vi "initialize_oscilloscope_chan1.vi"(0 "Range (0.001 S)":dbl=1.0 format="%#_13g", 1 "error in (no error)":errorcluster) -> (2 "VISA resource name out":refnum<visa-resource-name>, 3 "channels":i32[](array[numeric]), 4 "number":i32, 5 "error out":errorcluster)   [LabVIEW 2018]
doc: "This example shows how to configure multiple channels and acquire waveforms from multiple channels."
uses:
  <instrlib>/Agilent 2000 3000 X-Series/Agilent 2000 3000 X-Series.lvlib
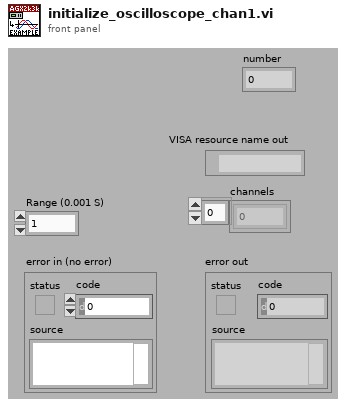
[diagram p1: front panel]
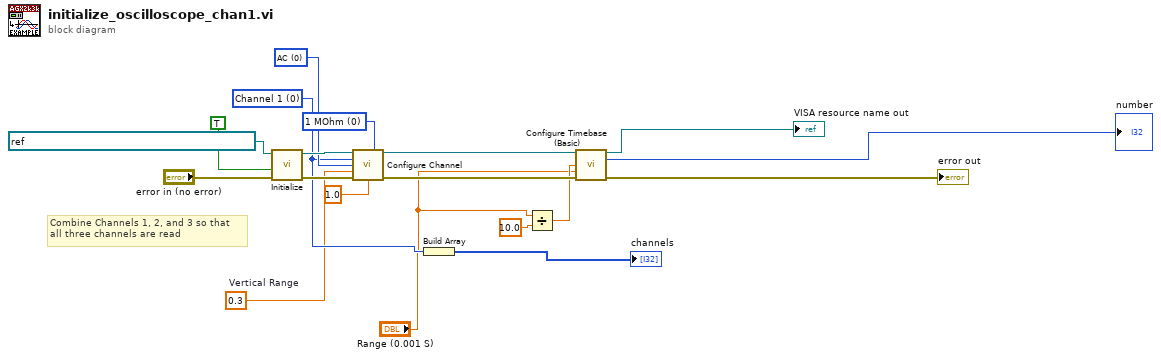
[diagram p0: block diagram]
diagram:
  w5 = 0 items=["1 MOhm", "50 Ohm"] ("Impedance (0: 1 MOhm)")
  w14 = 0 items=["AC", "DC", "Ground"] ("Vertical Coupling (1: DC)")
  w11 = 0 items=["Channel 1", "Channel 2", "Channel 3", "Channel 4"] ("Channel (0: Channel 1)")
  w8 = 0.3  # Vertical Range
  # "Combine Channels 1, 2, and 3 so that\nall three channels are read"
  n1 = call <instrlib>:"Initialize.vi"("error in (no error)"="error in (no error)", "Reset (True)"=TRUE, "VISA resource name"=refnum<visa-resource-name> "USB0::0x0957::0x1796::MY56272306::INSTR") -> ("error out"=w18:errorcluster, "VISA resource name out"=w17:refnum<visa-resource-name>)  [unwired: 2 in, 5 out]
  n2 = call <instrlib>:"Configure Channel.vi"("VISA resource name"=w17, "Impedance (0: 1 MOhm)"=w5, "Channel Name (0: Channel 1)"=w11, "Coupling (1: DC)"=w14, "Vertical Range (40.0 V)"=w8, "error in (no error)"=w18, "Probe Attenuation (1.0)"=1.0 ("Probe Attenuation (10.0)")) -> ("VISA resource name out"=w7:refnum<visa-resource-name>, "error out"=w6:errorcluster)  [unwired: 4 in, 3 out]
  n3 = Build Array(w11) -> (→"channels":i32[])
  n4 = Divide(x="Range (0.001 S)", y=10.0) -> (x/y=w3:dbl)
  n5 = call <instrlib>:"Configure Timebase (Basic).vi"("VISA resource name"=w7, "Scale (50 s/div)"=w3, "Range (0.001 S)"="Range (0.001 S)", "error in (no error)"=w6) -> ("VISA resource name out"=→"VISA resource name out":refnum<visa-resource-name>, "number"=→"number":i32, "error out"=→"error out":errorcluster)  [unwired: 5 in, 4 out]
